vi "single_trigger_setup.vi"(11 "Override in":T1) -> (3 "Override out":T1)   [LabVIEW 2013]
uses:
  ui_override_opts.ctl
panel:
  # "Set things up for single triggered non-averaged operation."
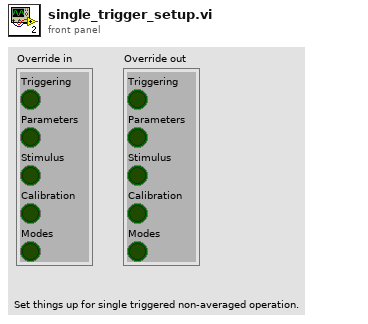
[diagram p1: front panel]
types:
  T1 = typedef "ui_override_opts.ctl" = cluster{"Triggering":bool, "Parameters":bool, "Stimulus":bool, "Calibration":bool, "Modes":bool}
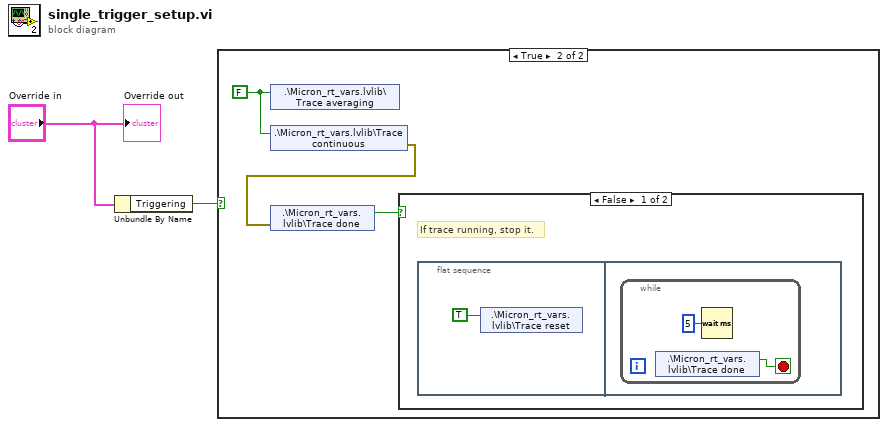
[diagram p0: block diagram]
diagram:
  n1 = Unbundle By Name("Override in") -> ("Triggering"=w2:bool)
  n2 = case shown="True" w2 {
    frame False {
    }
    frame True {
      w4 = FALSE ("Trace averaging")
      n3 = shared-variable ".\\Micron_rt_vars.lvlib\\Trace averaging"(w4) -> ()  [unwired: 2 out]
      n4 = shared-variable ".\\Micron_rt_vars.lvlib\\Trace continuous"(w4) -> (error out=w3:errorcluster)  [unwired: 1 out]
      n5 = shared-variable ".\\Micron_rt_vars.lvlib\\Trace done"(error in=w3) -> (w5:bool)  [unwired: 1 out]
      n6 = case shown="False" w5 {
        frame False {
          # "If trace running, stop it."
          n7 = flat-sequence {
            frame #0 {
              n8 = shared-variable ".\\Micron_rt_vars.lvlib\\Trace reset"(TRUE ("Start trace")) -> ()  [unwired: 2 out]
            }
            frame #1 {
              n9 = while {
                stop <- w7 stop-if-true
                n10 = shared-variable ".\\Micron_rt_vars.lvlib\\Trace done"() -> (w7:bool)  [unwired: 2 out]
                n11 = Wait (ms)(milliseconds to wait=u32 5) -> ()  [unwired: 1 out]
              }
            }
          }
        }
        frame True {
        }
      }
    }
  }
  "Override out" <- "Override in"
